vi "Launcher.vi"(11 "Error in":errorcluster caption="Error in (no error)") -> (15 "Error out":errorcluster)   [LabVIEW 2019]
doc: "<Developer>\nGPower\n10/6 2019"
uses:
  Diplom Controller/Diplom Controller/Diplom Controller.lvclass
  C:/Program Files (x86)/National Instruments/LabVIEW 2019/vi.lib/ActorFramework/Actor/Actor.lvclass
  <vilib>/ActorFramework/Actor/Actor.lvclass
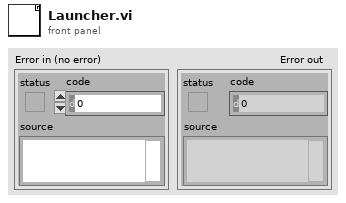
[diagram p1: front panel]
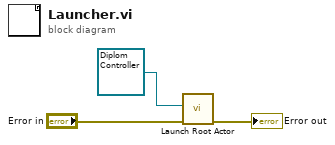
[diagram p0: block diagram]
diagram:
  n1 = call <vilib>:"Launch Root Actor.vi"("error in (no error)"="Error in", "Actor"=refnum<class "Diplom Controller.lvclass"> refnum ("Diplom Controller.lvlib:Diplom Controller.lvclass")) -> ("error out"=→"Error out":errorcluster)  [unwired: 8 in, 1 out]
